vi "set_binding_paths.vi"(8 "error in (no error)":errorcluster, 9 "OME header import string ref":refnum<k21>, 10 "notebook import string ref":refnum<k21>, 11 "DataCollectionDL090215 in":refnum<class "DataCollectionDL090215.lvclass">) -> (0 "error out":errorcluster, 3 "DataCollectionDL090215 out":refnum<class "DataCollectionDL090215.lvclass">)   [LabVIEW 2010, in "DataCollectionDL090215.lvclass"]
doc: "This method sets the data-binding paths (for the Shared Variable Enginge) for the import strings for the OME header and the notebook. By binding the two import strings to shared variables populated by software on some other computer, additional information for the file header or the notebook can be imported."
uses:
  DataCollectionDL090215.lvclass
  DataCollectionDL091104Scaffold/DataCollectionDL091104Scaffold/DataCollectionDL091104Scaffold.lvclass
  DataCollectionDL090215.lvclass/DataCollectionDL090215.ctl
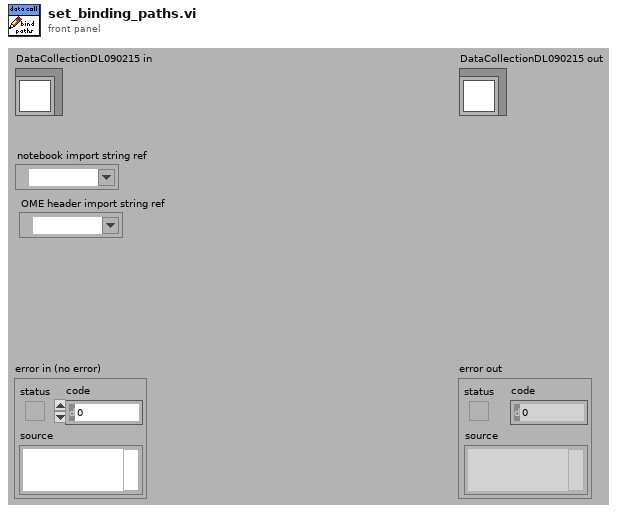
[diagram p1: front panel]
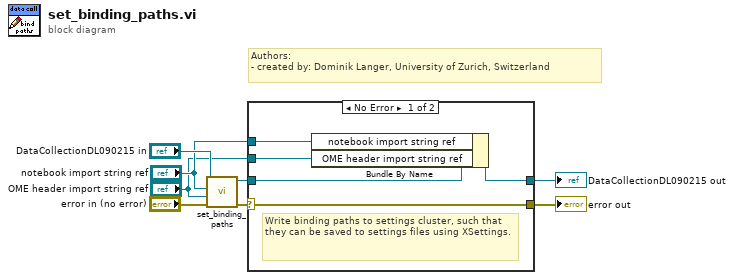
[diagram p0: block diagram]
diagram:
  # "Authors: \n- created by: Dominik Langer, University of Zurich, Switzerland"
  n1 = call-parent "set_binding_paths.vi"("error in (no error)"="error in (no error)", "OME header import string ref"="OME header import string ref", "notebook import string ref"="notebook import string ref", "DataCollectionDL091104Scaffold in"="DataCollectionDL090215 in") -> ("error out"=w5:errorcluster, "DataCollectionDL091104Scaffold out"=w6:refnum<class "DataCollectionDL090215.lvclass">)  [unwired: 6 in]
  n2 = case shown="No Error" w5 {
    selector: w5 -> [w12 w14]
    tunnel: w6 -> [w13 w15]
    tunnel: [w12 w14] -> w4
    tunnel: [w11 w15] -> w3
    tunnel: "notebook import string ref" -> [w10 _]
    tunnel: "OME header import string ref" -> [w9 _]
    frame No Error {
      # "Write binding paths to settings cluster, such that they can be saved to settings files using XSettings."
      n3 = Bundle By Name(cluster=w13, "notebook import string ref"=w10, "OME header import string ref"=w9) -> (w11:refnum<class "DataCollectionDL090215.lvclass">)
    }
    frame Error {
    }
  }
  "error out" <- w4
  "DataCollectionDL090215 out" <- w3
